vi "YearToFirstDayW01.vi"(10 "year":i32) -> (2 "First Day of W01":timestamp)   [LabVIEW 2018, in "DateTime.ISO8601.lvclass"]
uses:
  DateTime.ISO8601.lvclass
  <vilib>/Utility/miscctls.llb/LVDateTimeRec.ctl
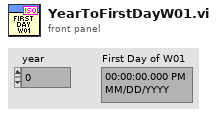
[diagram p1: front panel]
types:
  T1 = typedef "LVDateTimeRec.ctl" = cluster{"fractional second":dbl, "second":i32, "minute":i32, "hour":i32, "day of month":i32, "month":i32, "year":i32, "day of week":i32, "day of year":i32, "DST":i32}
  T2 = typedef "ISO Day -- enum.ctl" = enum16{"Monday", "Tuesday", "Wednesday", "Thursday", "Friday", "Saturday", "Sunday"}
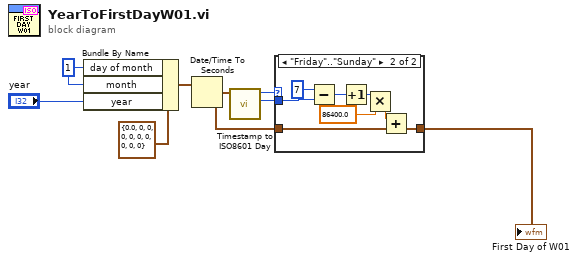
[diagram p0: block diagram]
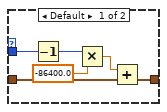
[diagram p2: hidden frame]
diagram:
  w2 = 1 ("day of month")
  n1 = Bundle By Name(cluster=T1 {"fractional second"=0.0, "second"=0, "minute"=0, "hour"=0, "day of month"=0, "month"=0, "year"=0, "day of week"=0, "day of year"=0, "DST"=0} ("date time rec"), "day of month"=w2, "month"=w2, "year"="year") -> (w3:T1)
  n2 = Date/Time To Seconds(2:w3) -> (0:w5:timestamp)  [unwired: 1 in]
  n3 = call "Timestamp to ISO8601 Day.vi"("Timestamp (now)"=w5) -> ("ISO Weekday"=w4:i32, "ISO Day"=w6:T2)  [unwired: 8 in, 1 out]
  n4 = case shown="\"Friday\"..\"Sunday\"" w6 {
    tunnel: w5 -> [w14 w22]
    tunnel: [w13 w21] -> w8
    tunnel: w4 -> [w11 w19]
    frame Default {
      n5 = Decrement(x=w11) -> (x-1=w10:i32)
      n6 = Multiply(x=w10, y=-86400.0 ("x")) -> (x*y=w12:dbl)
      n7 = Add(x=w12, y=w14) -> (x+y=w13:timestamp)
    }
    frame "Friday".."Sunday" {
      n8 = Subtract(x=7, y=w19) -> (x-y=w17:i32)
      n9 = Increment(x=w17) -> (x+1=w16:i32)
      n10 = Multiply(x=w16, y=86400.0 ("x")) -> (x*y=w20:dbl)
      n11 = Add(x=w20, y=w22) -> (x+y=w21:timestamp)
    }
  }
  "First Day of W01" <- w8
